vi "Benchmark mupExpr_eval_bulk.vi"(8 "error in (no error)":errorcluster, 10 "Iterations":i32=100000, 11 "Expression":string="5*x^2+2*x+20") -> (0 "error out":errorcluster, 2 "x":dbl[](array[numeric]), 3 "y":dbl[](array[numeric]), 5 "dt average":dbl)   [LabVIEW 2015]
uses:
  mupExpr/mupExpr.lvclass
  mupExpr/mupExpr.lvclass/mupExpr.ctl
  mupLib/mupEvalBulk.vi
  mupLib/mupSetVarValue_Array.vi
  mupLib/mupCheckError.vi
  mupLib/mupLibPath.vi
  <vilib>/Utility/error.llb/Error Cluster From Error Code.vi
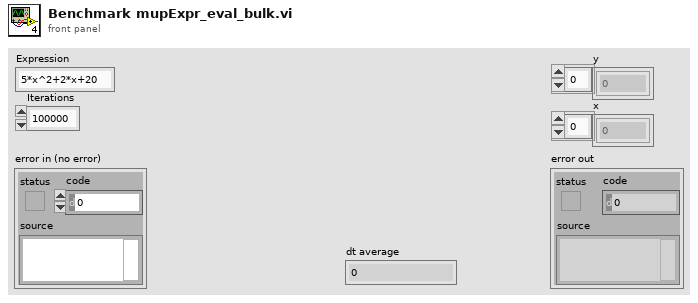
[diagram p1: front panel]
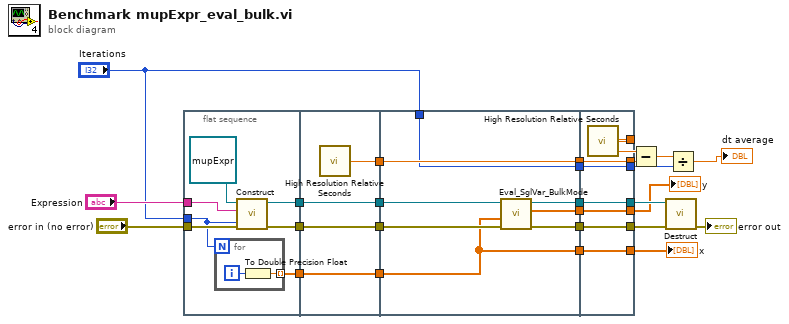
[diagram p0: block diagram]
diagram:
  n1 = flat-sequence {
    tunnel: [w30] -> w7
    tunnel: [w31] -> w6
    tunnel: "Expression" -> [w33]
    tunnel: "error in (no error)" -> [w32]
    tunnel: "Iterations" -> [w29]
    tunnel: [w28] -> w1
    tunnel: [w39] -> w21
    tunnel: [w38] -> w20
    tunnel: [w37] -> w14
    tunnel: w7 -> [w39]
    tunnel: w6 -> [w38]
    tunnel: [w36] -> w2
    tunnel: w1 -> [w36]
    tunnel: w21 -> [w47]
    tunnel: w20 -> [w46]
    tunnel: [w45] -> w19
    tunnel: [w44] -> w18
    tunnel: [w43] -> w17
    tunnel: [w40] -> w16
    tunnel: [w42] -> w15
    tunnel: w14 -> [w42]
    tunnel: "Iterations" -> [w41]
    tunnel: [w41] -> w9
    tunnel: w2 -> [w40]
    tunnel: [w51] -> w23
    tunnel: [w52] -> w24
    tunnel: [w53] -> w25
    tunnel: [w54] -> w26
    tunnel: w19 -> [w54]
    tunnel: w18 -> [w53]
    tunnel: w17 -> [w52]
    tunnel: w16 -> [w51]
    tunnel: [w50] -> w12
    tunnel: w15 -> [w50]
    tunnel: [w49] -> w13
    tunnel: [w48] -> w10
    tunnel: w9 -> [w48]
    frame #0 {
      n2 = for {
        N: w29 -> [_]
        tunnel: [w34] -> w28 mode=indexing
        i -> [w35]
        n3 = To Double Precision Float(number=w35) -> (double precision float=w34:dbl)
      }
      n4 = call-dynamic "Construct.vi"("Bulk Size (1)"=w29, "error in (no error)"=w32, "Expression"=w33, "muExpr in"=refnum<class "mupExpr.lvclass"> refnum) -> ("error out"=w31:errorcluster, "mupExpr out"=w30:refnum<class "mupExpr.lvclass">)  [unwired: 4 in, 2 out]
    }
    frame #1 {
      n5 = call <vilib>:"High Resolution Relative Seconds.vi"() -> ("relative seconds"=w37:dbl)
    }
    frame #2 {
      n6 = call "Eval_SglVar_BulkMode.vi"("error in (no error)"=w46, "varValue"=w40, "muExpr in"=w47) -> ("error out"=w44:errorcluster, "Result"=w43:dbl[], "muExpr out"=w45:refnum<class "mupExpr.lvclass">)  [unwired: 6 in]
    }
    frame #3 {
      n7 = call <vilib>:"High Resolution Relative Seconds.vi"() -> ("relative seconds"=w49:dbl)
    }
  }
  n8 = Subtract(x=w13, y=w12) -> (x-y=w11:dbl)
  n9 = call-dynamic "Destruct.vi"("error in (no error)"=w25, "muExpr in"=w26) -> ("error out"=→"error out":errorcluster)  [unwired: 9 in]
  n10 = Divide(x=w11, y=w10) -> (x/y=→"dt average":dbl)
  "y" <- w24
  "x" <- w23
